vi "Drive.vi"() -> ()   [LabVIEW 2018]
uses:
  <vilib>/Rock Robotics/WPI/ThirdParty/Phoenix-LabVIEW/Motor Controller/Controls/CTRE_Phoenix_MotorControl_StatusFrameEnhanced.ctl
  DriveLoopEnum.ctl
  2019_Robot_Code/Subsystems/Drive/driveShifterEnum.ctl
  <vilib>/Rock Robotics/WPI/ThirdParty/Phoenix-LabVIEW/Motor Controller/Controls/CTRE_Phoenix_MotorControl_ControlMode.ctl
  <vilib>/Rock Robotics/WPI/Utilities/WPI_GetSetVariantRefNum.vi
  <vilib>/Rock Robotics/WPI/ThirdParty/Phoenix-LabVIEW/Motor Controller/Get/CTRE_Phoenix_MotorController_GetQuadratureData.vi
  <vilib>/Rock Robotics/WPI/ThirdParty/Phoenix-LabVIEW/Pigeon IMU/CTRE_PigeonIMU_GetFusedHeading.vi
panel:
  in  "IMU PID (P)":dbl
  in  "Feed Forward":dbl
  out "Motion Magic Distance (Raw Units)":dbl
  in  "Motion Magic Distance (Inches)":dbl
  out "Right Drive Encoder":i32(graph)
  out "Left Drive Encoder":i32(graph)
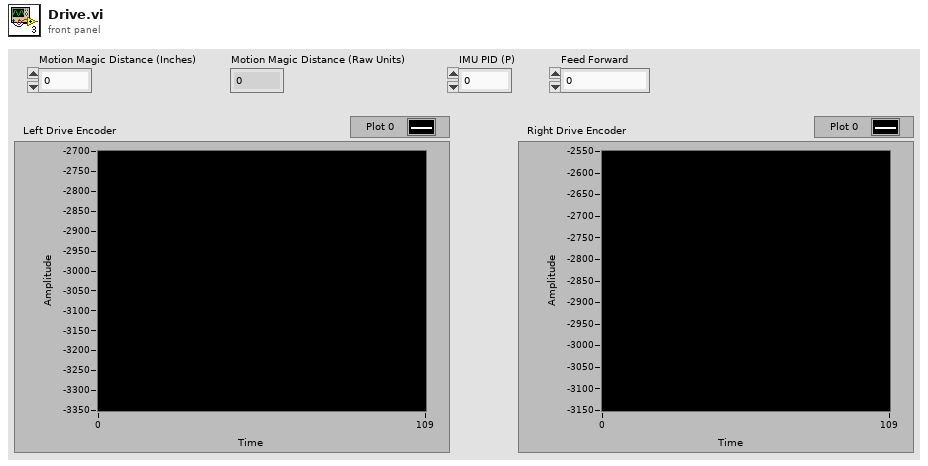
[diagram p1: front panel]
types:
  T1 = typedef "CTRE_PigeonIMU_DeviceRef.ctl" = cluster{"DeviceStatus":errorcluster, "Device Number":u8, "Type":T2, "Device ID":u32, "Handle":u64, "UsageFrame":u32, "Library Path":path}
  T2 = typedef "CTRE_PigeonIMU_ConnectionType.ctl" = u32
  T3 = typedef "driveShifterEnum.ctl" = enum16{"Low", "High"}
  T4 = enum16{"Inches -> Sensor Units", "Sensor Units -> Inches"}
  T5 = typedef "DriveLoopEnum.ctl" = enum16{"Manual", "Motion Magic", "Reset Encoders", "Feed Forward Calculation"}
  T6 = typedef "CTRE_Phoenix_MotorControl_StatusFrameEnhanced.ctl" = u16
  T7 = typedef "WPI_MotorControlDeviceRef.ctl" = cluster{"DeviceStatus":errorcluster, "Type":T8, "PWM":cluster{"PWM Channel":T9, "DeadBand":T10}, "CAN":cluster{"Device Number":u8, "SetOutput VI Ref":variant, "GetOutput VI Ref":variant, "Enable VI Ref":variant, "Disable VI Ref":variant, "Data":variant}, "Invert":bool, "DIO PWM":cluster{"PWM \"Enable\" Channel":T9, "DIOChannel":T11, "PWM Rate":dbl}}
  T8 = typedef "WPI_MotorControlType.ctl" = enum16{"PWM", "CAN", "DIO PWM"}
  T9 = typedef "FPGA_DIOPWMChannel.ctl" = enum8{"PWM 0", "PWM 1", "PWM 2", "PWM 3", "PWM 4", "PWM 5", "PWM 6", "PWM 7", "PWM 8", "PWM 9", "PWM MXP 0", "PWM MXP 1", "PWM MXP 2", "PWM MXP 3", "PWM MXP 4", "PWM MXP 5", "PWM MXP 6", "PWM MXP 7", "PWM MXP 8", "PWM MXP 9", "Invalid"}
  T10 = typedef "WPI_PWMDeadband.ctl" = cluster{"Name":string, "maxPositivePwm":i32, "minPositivePwm":i32, "centerPwm":i32, "maxNegativePwm":i32, "minNegativePwm":i32, "angularRange":u16}
  T11 = typedef "FPGA_DIOChannel.ctl" = enum8{"DIO 0", "DIO 1", "DIO 2", "DIO 3", "DIO 4", "DIO 5", "DIO 6", "DIO 7", "DIO 8", "DIO 9", "DIO MXP 0", "DIO MXP 1", "DIO MXP 2", "DIO MXP 3", "DIO MXP 4", "DIO MXP 5", "DIO MXP 6", "DIO MXP 7", "DIO MXP 8", "DIO MXP 9", "DIO MXP 10", "DIO MXP 11", "DIO MXP 12", "DIO MXP 13", "DIO MXP 14", "DIO MXP 15", "SPI Port CS1", "SPI Port CS2", "SPI Port CS3", "SPI Port MISO", "SPI Port MOSI", "Invalid"}
  T12 = typedef "WPI_JoystickDevRef.ctl" = cluster{"Device":T13}
  T13 = typedef "WPI_JoystickDeviceEnum.ctl" = enum16{"USB 0", "USB 1", "USB 2", "USB 3", "USB 4", "USB 5"}
  T14 = typedef "CTRE_Phoenix_MotorControl_ControlMode.ctl" = u16
  T15 = enum16{"DemandType_Neutral", "DemandType_AuxPID", "DemandType_ArbitraryFeedForward"}
  T16 = cluster{"Heading":dbl, "Valid?":bool, "Fusing?":bool}
  T17 = typedef "ConstantsControl.ctl" = cluster{"Drive Constants":cluster{"Minumum Feed Forward":dbl}}
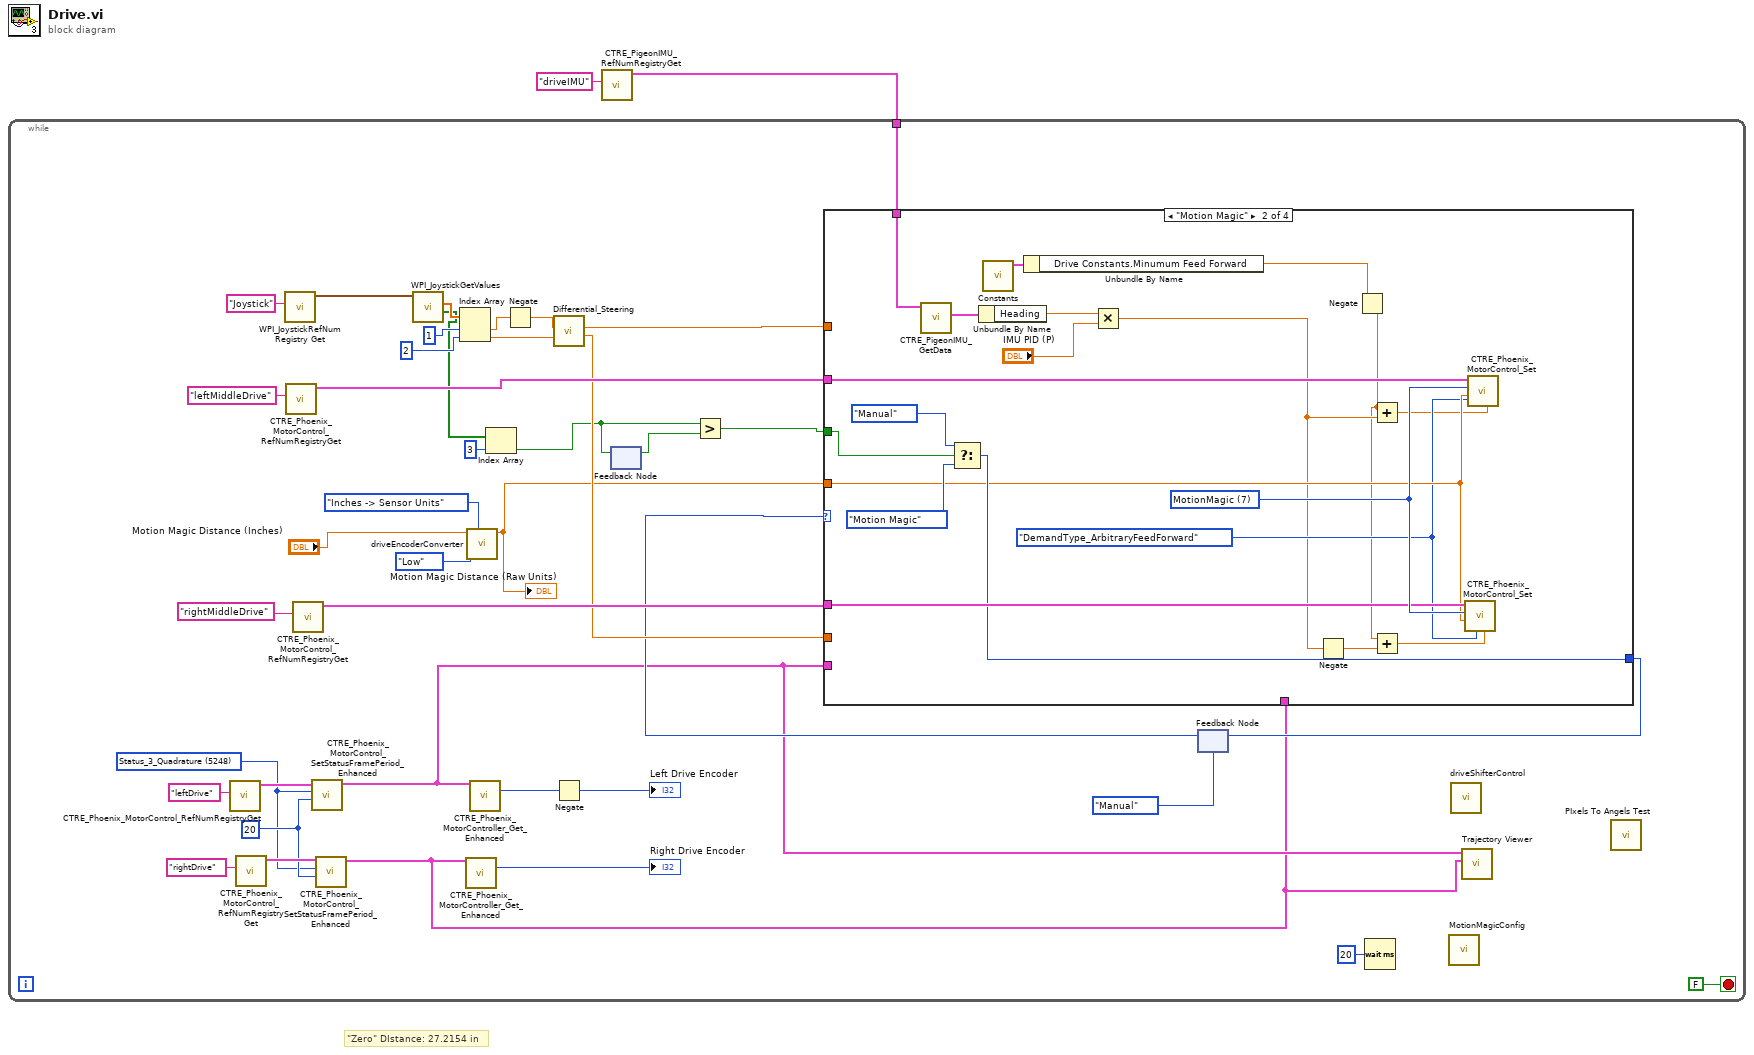
[diagram p0: block diagram]
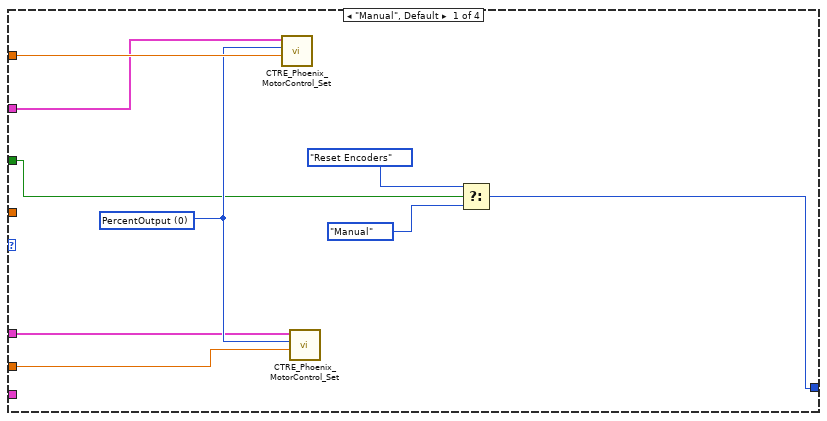
[diagram p2: hidden frame]
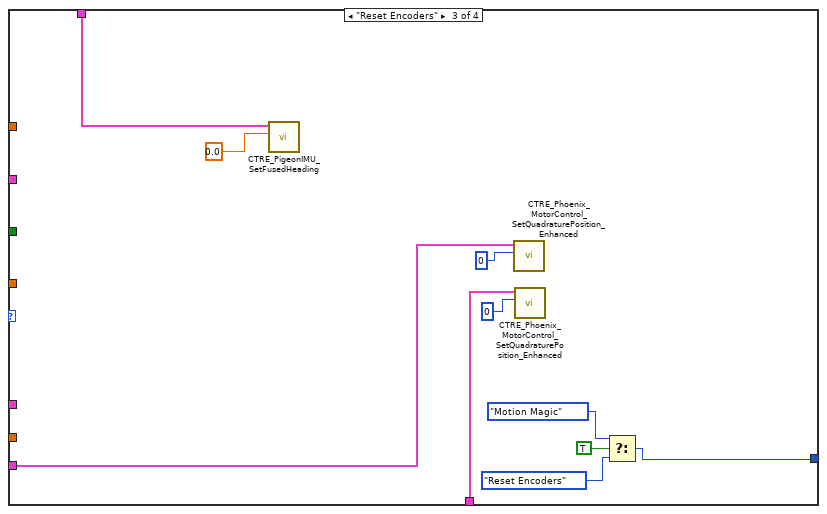
[diagram p3: hidden frame]
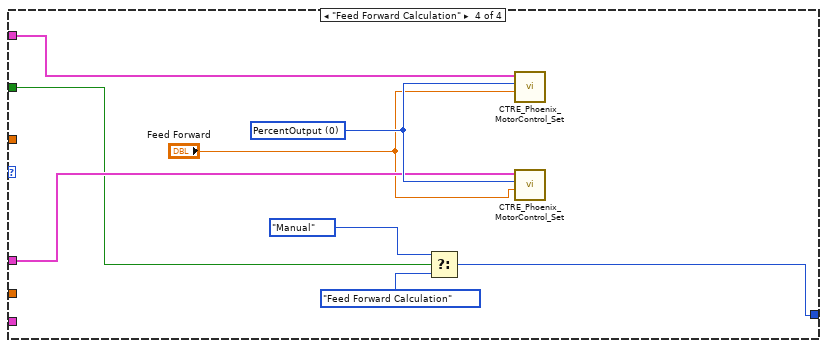
[diagram p4: hidden frame]
diagram:
  # "\"Zero\" DIstance: 27.2154 in"
  n1 = call <vilib>:"CTRE_PigeonIMU_RefNumRegistryGet.vi"("refnum name"="driveIMU") -> ("PigeonIMUDevRef"=w1:T1)  [unwired: 9 in, 1 out]
  n2 = while {
    tunnel: w1 -> [w3]
    stop <- FALSE stop-if-true
    w31 = T6 5248 items=["Status_1_General"=5120, "Status_2_Feedback0"=5184, "Status_3_Quadrature"=5248, "Status_4_AinTempVbat"=5312, "Status_6_Misc"=5440, "Status_7_CommStatus"=5504, "Status_8_PulseWidth"=5568, "Status_9_MotProfBuffer"=5632, "Status_10_MotionMagic"=5696, "Status_11_UartGadgeteer"=5760, "Status_12_Feedback1"=5824, "Status_13_Base_PIDF0"=5888, "Status_14_Turn_PIDF1"=5952, "Status_15_FirmwareApiStatus"=6016] ("Status Frame")
    w32 = 20 ("periodMs")
    n3 = call <vilib>:"CTRE_Phoenix_MotorControl_RefNumRegistryGet.vi"("refnum name"="leftDrive") -> ("PhoenixMotorControlDevRef"=w33:T7)  [unwired: 9 in, 1 out]
    n4 = call <vilib>:"CTRE_Phoenix_MotorControl_RefNumRegistryGet.vi"("refnum name"="rightDrive") -> ("PhoenixMotorControlDevRef"=w34:T7)  [unwired: 9 in, 1 out]
    n5 = call <vilib>:"WPI_JoystickRefNum Registry Get.vi"("refnum name"="Joystick") -> ("JoystickDevRef"=w41:T12)  [unwired: 9 in, 1 out]
    n6 = call <vilib>:"CTRE_Phoenix_MotorControl_RefNumRegistryGet.vi"("refnum name"="leftMiddleDrive") -> ("PhoenixMotorControlDevRef"=w38:T7)  [unwired: 9 in, 1 out]
    n7 = call <vilib>:"CTRE_Phoenix_MotorControl_RefNumRegistryGet.vi"("refnum name"="rightMiddleDrive") -> ("PhoenixMotorControlDevRef"=w37:T7)  [unwired: 9 in, 1 out]
    n8 = call <vilib>:"CTRE_Phoenix_MotorControl_SetStatusFramePeriod_Enhanced.vi"("periodMs"=w32, "Status Frame"=w31, "PhoenixMotorControlDevRef"=w33) -> ("PhoenixMotorControlDevRef"=w6:T7)  [unwired: 7 in, 1 out]
    n9 = call <vilib>:"CTRE_Phoenix_MotorControl_SetStatusFramePeriod_Enhanced.vi"("periodMs"=w32, "Status Frame"=w31, "PhoenixMotorControlDevRef"=w34) -> ("PhoenixMotorControlDevRef"=w5:T7)  [unwired: 7 in, 1 out]
    n10 = call <vilib>:"WPI_JoystickGetValues.vi"("JoystickDevRef"=w41) -> ("Buttons"=w19:bool[], "Axes"=w27:dbl[])  [unwired: 6 in, 3 out]
    n11 = Index Array(array=w27, index #1=1 ("index"), index #2=2 ("index")) -> (element #1=w28:dbl, element #2=w26:dbl)
    n12 = call-poly <vilib>:"CTRE_Phoenix_MotorController_Get_Enhanced.vi"("PhoenixMotorControlDevRef"=w5) -> ("Quadrature Position"=→"Right Drive Encoder":i32)  [unwired: 11 in, 3 out]
    n13 = call "driveEncoderConverter.vi"("Conversion Direction"=T4."Inches -> Sensor Units", "Gear Setting"=driveShifterEnum."Low", "Input"="Motion Magic Distance (Inches)") -> ("Output"=w7:dbl)  [unwired: 8 in]
    "Motion Magic Distance (Raw Units)" <- w7
    n14 = call-poly <vilib>:"CTRE_Phoenix_MotorController_Get_Enhanced.vi"("PhoenixMotorControlDevRef"=w6) -> ("Quadrature Position"=w23:i32)  [unwired: 11 in, 3 out]
    n15 = Index Array(array=w19, index=3) -> (element=w16:bool)
    n16 = Negate(x=w28) -> (-x=w20:dbl)
    n17 = call <userlib>:"Differential_Steering.vi"("Steer"=w26, "Base"=w20) -> ("Right"=w25:dbl, "Left"=w24:dbl)  [unwired: 4 in]
    n18 = Negate(x=w23) -> (-x=→"Left Drive Encoder":i32)
    n19 = feedback #1() -> (w15:bool)  [unwired: 1 in]
    n20 = feedback-in #1(w16) -> ()
    n21 = Greater?(x=w16, y=w15) -> (0:w17:bool)
    n22 = feedback #2(DriveLoopEnum."Manual" ("Enum")) -> (w12:T5)
    n23 = case shown="\"Motion Magic\"" w12 {
      tunnel: w25 -> [w51 _ _ _]
      tunnel: w24 -> [w50 _ _ _]
      tunnel: w38 -> [w48 w70 _ w88]
      tunnel: w37 -> [w47 w69 _ w87]
      tunnel: w6 -> [_ _ w81 _]
      tunnel: w5 -> [_ _ w80 _]
      tunnel: [w44 w65 w77 w83] -> w14
      tunnel: w17 -> [w43 w68 _ w82]
      tunnel: w7 -> [_ w64 _ _]
      tunnel: w3 -> [_ w60 w73 _]
      frame "Manual", Default {
        w49 = T14 0 items=["PercentOutput"=0, "Position"=1, "Velocity"=2, "Current"=3, "Follower"=5, "MotionProfile"=6, "MotionMagic"=7, "MotionProfileArc"=10, "Disabled"=15] ("Control Mode")
        n24 = call <vilib>:"CTRE_Phoenix_MotorControl_Set.vi"("Output"=w50, "Control Mode"=w49, "PhoenixMotorControlDevRef"=w48) -> ()  [unwired: 7 in, 2 out]
        n25 = call <vilib>:"CTRE_Phoenix_MotorControl_Set.vi"("Output"=w51, "Control Mode"=w49, "PhoenixMotorControlDevRef"=w47) -> ()  [unwired: 7 in, 2 out]
        n26 = Select(t=DriveLoopEnum."Reset Encoders" ("Enum"), s=w43, f=DriveLoopEnum."Manual" ("Enum")) -> (s? t:f=w44:T5)
      }
      frame "Motion Magic" {
        w63 = T15."DemandType_ArbitraryFeedForward" ("DemandType")
        w71 = T14 7 items=["PercentOutput"=0, "Position"=1, "Velocity"=2, "Current"=3, "Follower"=5, "MotionProfile"=6, "MotionMagic"=7, "MotionProfileArc"=10, "Disabled"=15] ("Control Mode")
        n27 = call-poly <vilib>:"CTRE_PigeonIMU_GetData.vi"("PigeonIMUDevRef"=w60) -> ("Fused Heading"=w59:T16)  [unwired: 8 in, 2 out]
        n28 = Select(t=DriveLoopEnum."Manual" ("Enum"), s=w68, f=DriveLoopEnum."Motion Magic" ("Enum")) -> (s? t:f=w65:T5)
        n29 = Unbundle By Name(w59) -> ("Heading"=w58:dbl)
        n30 = call "Constants.vi"() -> ("Cluster"=w62:T17)  [unwired: 11 in]
        n31 = Unbundle By Name(w62) -> ("Drive Constants.Minumum Feed Forward"=w61:dbl)
        n32 = Multiply(x=w58, y="IMU PID (P)") -> (x*y=w54:dbl)
        n33 = Negate(x=w54) -> (-x=w53:dbl)
        n34 = Negate(x=w61) -> (-x=w52:dbl)
        n35 = Add(x=w52, y=w54) -> (x+y=w56:dbl)
        n36 = Add(x=w52, y=w53) -> (x+y=w55:dbl)
        n37 = call <vilib>:"CTRE_Phoenix_MotorControl_Set.vi"("Demand1"=w55, "DemandType"=w63, "Output"=w64, "Control Mode"=w71, "PhoenixMotorControlDevRef"=w69) -> ()  [unwired: 5 in, 2 out]
        n38 = call <vilib>:"CTRE_Phoenix_MotorControl_Set.vi"("Demand1"=w56, "DemandType"=w63, "Output"=w64, "Control Mode"=w71, "PhoenixMotorControlDevRef"=w70) -> ()  [unwired: 5 in, 2 out]
      }
      frame "Reset Encoders" {
        n39 = call <vilib>:"CTRE_PigeonIMU_SetFusedHeading.vi"("Value"=0.0, "PigeonIMUDevRef 2"=w73) -> ()  [unwired: 8 in, 2 out]
        n40 = call <vilib>:"CTRE_Phoenix_MotorControl_SetQuadraturePosition_Enhanced.vi"("New Position"=0, "PhoenixMotorControlDevRef"=w81) -> ()  [unwired: 8 in, 2 out]
        n41 = call <vilib>:"CTRE_Phoenix_MotorControl_SetQuadraturePosition_Enhanced.vi"("New Position"=0, "PhoenixMotorControlDevRef"=w80) -> ()  [unwired: 8 in, 2 out]
        n42 = Select(t=DriveLoopEnum."Motion Magic" ("Enum"), s=TRUE, f=DriveLoopEnum."Reset Encoders" ("Enum")) -> (s? t:f=w77:T5)
      }
      frame "Feed Forward Calculation" {
        w89 = T14 0 items=["PercentOutput"=0, "Position"=1, "Velocity"=2, "Current"=3, "Follower"=5, "MotionProfile"=6, "MotionMagic"=7, "MotionProfileArc"=10, "Disabled"=15] ("Control Mode")
        n43 = Select(t=DriveLoopEnum."Manual" ("Enum"), s=w82, f=DriveLoopEnum."Feed Forward Calculation" ("Enum")) -> (s? t:f=w83:T5)
        n44 = call <vilib>:"CTRE_Phoenix_MotorControl_Set.vi"("Output"="Feed Forward", "Control Mode"=w89, "PhoenixMotorControlDevRef"=w88) -> ()  [unwired: 7 in, 2 out]
        n45 = call <vilib>:"CTRE_Phoenix_MotorControl_Set.vi"("Output"="Feed Forward", "Control Mode"=w89, "PhoenixMotorControlDevRef"=w87) -> ()  [unwired: 7 in, 2 out]
      }
    }
    n46 = feedback-in #2(w14) -> ()
    n47 = Wait (ms)(milliseconds to wait=u32 20) -> ()  [unwired: 1 out]
    n48 = call "MotionMagicConfig.vi"() -> ()  [unwired: 12 in]
    n49 = call "driveShifterControl.vi"() -> ()  [unwired: 12 in]
    n50 = call "Trajectory Viewer.vi"("RightDrive"=w5, "LeftDrive"=w6) -> ()  [unwired: 10 in]
    n51 = call "PIxels To Angels Test.vi"() -> ()  [unwired: 12 in]
  }
